vi "Get Empty Row.vi"(8 "error in (no error)":errorcluster) -> (0 "error out":errorcluster, 3 "Empty Row":string[](array[string]))   [LabVIEW 2020, in "Astemes_CSVReportPlugin.lvlib" / "TestStand Result Handler.lvclass"]
uses:
  TestStand Result Handler.lvclass
  Columns.ctl
  9db46f2e-3e16-4312-b9c5-d87a26773705.vi
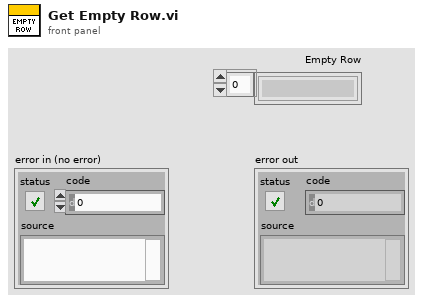
[diagram p1: front panel]
types:
  T1 = typedef "Astemes_CSVReportPlugin.lvlib/TestStand Result Handler.lvclass/Columns.ctl" = enum16{"StepName", "Result", "LowerLimit", "ComparisonTypeLow", "Measurement", "ComparisonTypeHigh", "UpperLimit", "ReportText", "StepType"}
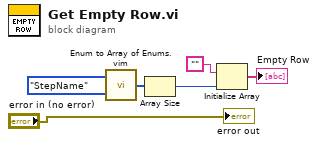
[diagram p0: block diagram]
diagram:
  n1 = call "Enum to Array of Enums.vim"("enum"=Columns."StepName" ("Column")) -> ("array of enums"=w5:T1[])
  n2 = Array Size(array=w5) -> (size(s)=w3:i32)
  n3 = Initialize Array("", w3) -> (→"Empty Row":string[])
  "error out" <- "error in (no error)"
